vi "Remove Single Wheel from Steering Frame.vi"(8 "error in (no error)":errorcluster, 10 "wheel index":i32, 11 "steering frame in":refnum<class "NI_Robotics_Steering Frame.lvclass">) -> (0 "error out":errorcluster, 1 "found?":bool, 2 "removed wheel":refnum<class "NI_Robotics_Wheel.lvclass">, 3 "steering frame out":refnum<class "NI_Robotics_Steering Frame.lvclass">, 4 "frame angle (rad)":dbl, 5 "y position":dbl, 7 "x position":dbl)   [LabVIEW 2017, in "NI_Robotics_Steering Frame.lvclass"]
doc: "Removes the wheel or wheels you specify from <B>steering frame in</B>. You must manually select the polymorphic instance to use."
uses:
  <vilib>/robotics/Steering/Steering Frame/NI_Robotics_Steering Frame.lvclass
  <vilib>/robotics/Steering/Wheel/NI_Robotics_Wheel.lvclass
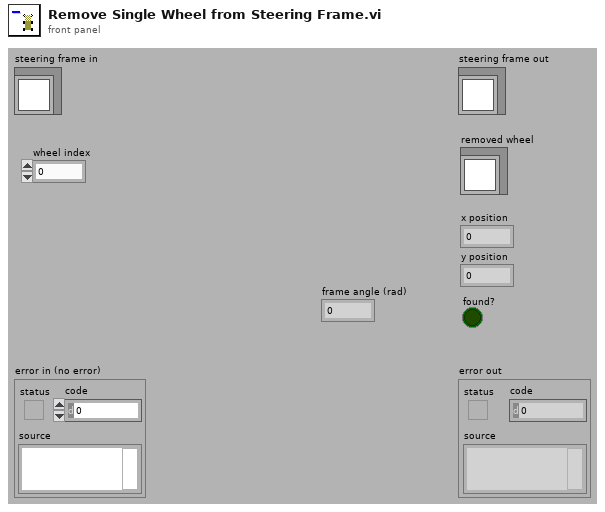
[diagram p1: front panel]
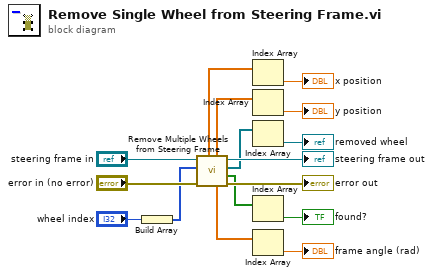
[diagram p0: block diagram]
diagram:
  n1 = Build Array("wheel index") -> (w11:i32[])
  n2 = call <vilib>:"Remove Multiple Wheels from Steering Frame.vi"("error in (no error)"="error in (no error)", "wheel indexes"=w11, "steering frame in"="steering frame in") -> ("error out"=→"error out":errorcluster, "found?"=w2:bool[], "removed wheels"=w6:refnum<class "NI_Robotics_Wheel.lvclass">[], "steering frame out"=→"steering frame out":refnum<class "NI_Robotics_Steering Frame.lvclass">, "frame angles (rad)"=w4:dbl[], "y positions"=w8:dbl[], "x positions"=w10:dbl[])  [unwired: 2 in]
  n3 = Index Array(array=w10) -> (element=→"x position":dbl)  [unwired: 1 in]
  n4 = Index Array(array=w8) -> (element=→"y position":dbl)  [unwired: 1 in]
  n5 = Index Array(array=w6) -> (element=→"removed wheel":refnum<class "NI_Robotics_Wheel.lvclass">)  [unwired: 1 in]
  n6 = Index Array(array=w2) -> (element=→"found?":bool)  [unwired: 1 in]
  n7 = Index Array(array=w4) -> (element=→"frame angle (rad)":dbl)  [unwired: 1 in]
